vi "Check if configuration files exist.vi"(8 "error in (no error)":errorcluster, 11 "TemplateBase in":refnum<class "BMC.lvclass">) -> (0 "error out":errorcluster, 2 "configuration file exists?":bool, 3 "TemplateBase out":refnum<class "BMC.lvclass">)   [LabVIEW 2012, in "BMC.lvclass"]
doc: "Checks whether all required configuration files for the component exist."
uses:
  BMC.lvclass
  <vilib>/Distrio/Murmex/Murmex/Murmex.lvclass
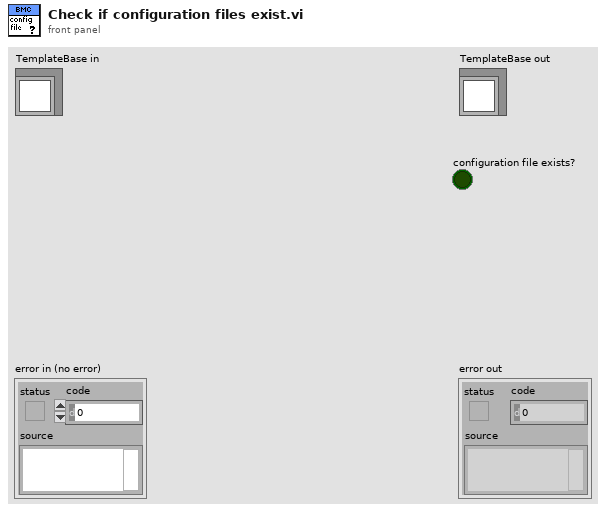
[diagram p1: front panel]
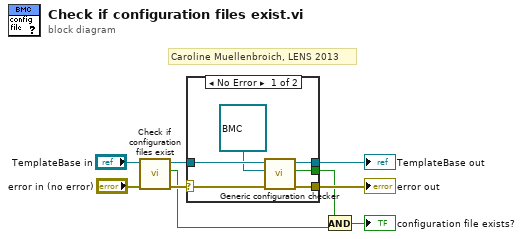
[diagram p0: block diagram]
diagram:
  # "Caroline Muellenbroich, LENS 2013"
  n1 = call-parent "Check if configuration files exist.vi"("error in (no error)"="error in (no error)", "MurmexBase in"="TemplateBase in") -> ("error out"=w7:errorcluster, "configuration file exists?"=w3:bool, "MurmexBase out"=w6:refnum<class "BMC.lvclass">)  [unwired: 7 in]
  n2 = case shown="No Error" w7 {
    selector: w7 -> [w15 w17]
    tunnel: [w13 w17] -> w5
    tunnel: [w11 w16] -> w4
    tunnel: w6 -> [w14 w16]
    tunnel: [w12 _] -> w1
    frame No Error {
      n3 = call <vilib>:"Generic configuration checker.vi"("error in (no error)"=w15, "inheritance level"=refnum<class "BMC.lvclass"> refnum ("Template.lvclass"), "Murmex in"=w14) -> ("error out"=w13:errorcluster, "configuration file exists?"=w12:bool, "Murmex out"=w11:refnum<class "BMC.lvclass">)  [unwired: 6 in]
    }
    frame Error {
    }
  }
  "error out" <- w5
  "TemplateBase out" <- w4
  n4 = And(x=w1, y=w3) -> (x .and. y?=→"configuration file exists?":bool)
